vi "File.Check if Exists, Small Icon.vi"(11 "Path":path) -> (2 "Exists":bool, 3 "Dup Path":path, 5 "Does Not Exist":bool)   [LabVIEW 2024]
uses:
  File Utils.lvlib
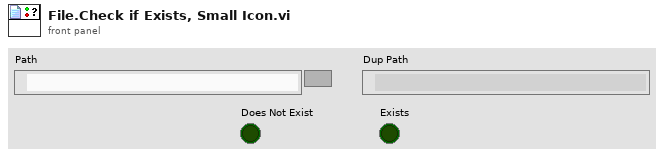
[diagram p1: front panel]
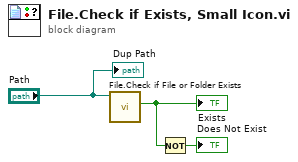
[diagram p0: block diagram]
diagram:
  n1 = call "File.Check if File or Folder Exists.vi"("Path"="Path") -> ("Exists"=w2:bool)  [unwired: 6 in, 4 out]
  "Exists" <- w2
  n2 = Not(x=w2) -> (.not. x?=→"Does Not Exist":bool)
  "Dup Path" <- "Path"
